vi "42_Overlay_Rectangle.vi"() -> ()   [LabVIEW 2018]
panel:
  in  "Stop":bool caption="Stop (F)"
  out "Image Out":T1(plugin-control)
  # "物件外框"
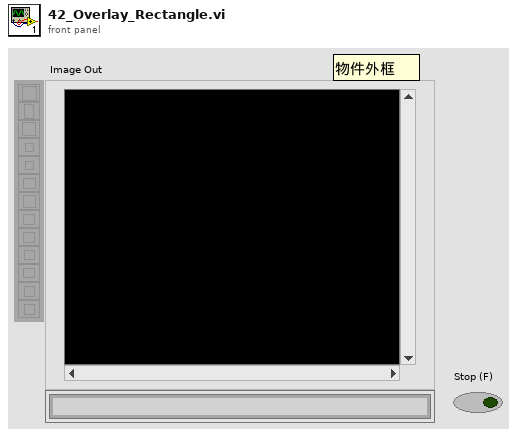
[diagram p1: front panel]
types:
  T1 = typedef "IMAQ Image.ctl" = refnum<image>
  T2 = cluster{"Left":dbl, "Top":dbl, "Right":dbl, "Bottom":dbl}
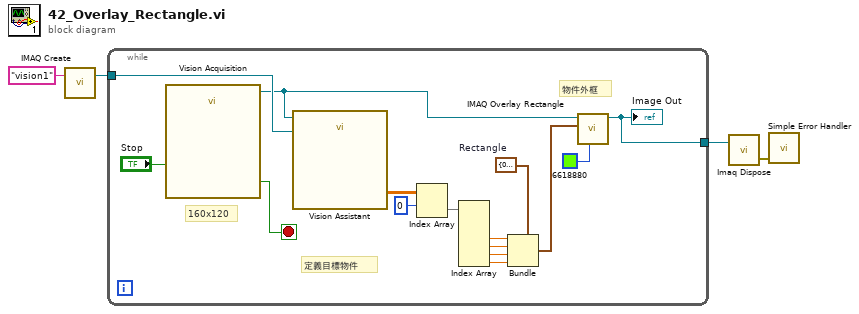
[diagram p0: block diagram]
diagram:
  n1 = call "IMAQ Create"("Image Name"="vision1") -> ("New Image"=w3:T1)  [unwired: 4 in, 1 out]
  n2 = while {
    tunnel: w3 -> [w9]
    tunnel: [w5] -> w1
    stop <- w18 stop-if-true
    w15 = T2 {"Left"=0.0, "Top"=0.0, "Right"=0.0, "Bottom"=0.0}  # Rectangle
    # "定義目標物件"
    # "物件外框"
    # "160x120"
    n3 = call "Vision Acquisition"("Stop (F)"="Stop") -> ("Image Out"=w8:T1, "Stopped"=w18:bool)  [unwired: 24 in, 1 out]
    n4 = call "Vision Assistant"("Image In"=w8, "Image Dst"=w9) -> ("Particle Measurements (Pixels) (Particle Analysis 1)"=w17:dbl[][])  [unwired: 22 in, 3 out]
    n5 = Index Array "Index Array"(array=w17, index (row)=0) -> (element=w16:dbl[])  [unwired: 1 in]
    n6 = Index Array "Index Array"(array=w16) -> (element #3=w14:dbl, element #4=w13:dbl, element #5=w12:dbl, element #6=w11:dbl)  [unwired: 6 in, 2 out]
    n7 = Bundle "Bundle"(cluster=w15, "Left"=w14, "Top"=w13, "Right"=w12, "Bottom"=w11) -> (w6:T2)
    n8 = call "IMAQ Overlay Rectangle"("Color"=u32 6618880, "Rectangle"=w6, "Image"=w8) -> ("Image Out"=w5:T1)  [unwired: 7 in, 1 out]
    "Image Out" <- w5
  }
  n9 = call "Imaq Dispose"("Image"=w1) -> ("error out"=w2:errorcluster)  [unwired: 5 in]
  n10 = call <vilib>:"Simple Error Handler.vi"("error in (no error)"=w2) -> ()  [unwired: 4 in, 5 out]
